vi "Write Epsilon.vi"(8 "error in (no error)":errorcluster, 10 "Epsilon":dbl, 11 "HG Observer in":refnum<class "HG Observer.lvclass">) -> (0 "error out":errorcluster, 3 "HG Observer out":refnum<class "HG Observer.lvclass">)   [LabVIEW 2014, in "Observer Library.lvlib" / "HG Observer.lvclass"]
uses:
  HG Observer.lvclass
  HG Observer.lvclass/HG Observer.ctl
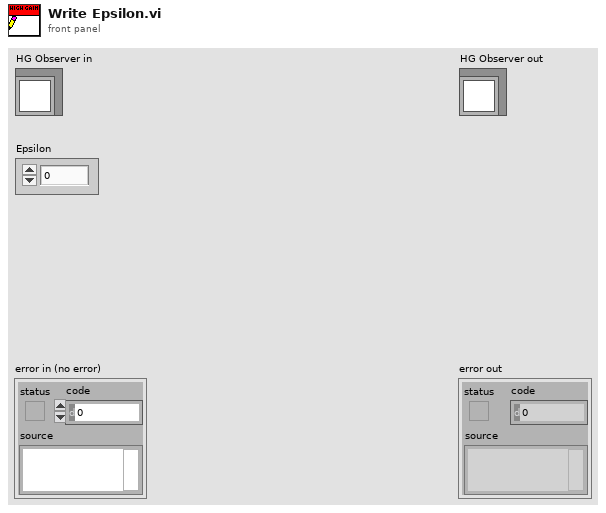
[diagram p1: front panel]
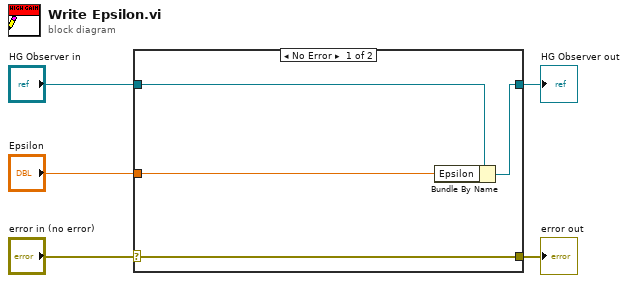
[diagram p0: block diagram]
diagram:
  n1 = case shown="No Error" "error in (no error)" {
    selector: "error in (no error)" -> [w9 w10]
    tunnel: [w9 w10] -> w4
    tunnel: [w7 w11] -> w2
    tunnel: "HG Observer in" -> [w8 w11]
    tunnel: "Epsilon" -> [w6 _]
    frame No Error {
      n2 = Bundle By Name(cluster=w8, "Epsilon"=w6) -> (w7:refnum<class "HG Observer.lvclass">)
    }
    frame Error {
    }
  }
  "error out" <- w4
  "HG Observer out" <- w2
